vi "Tick.vi"(7 "error in (no error)":errorcluster) -> (5 "error out":errorcluster, 11 "seconds":dbl)   [LabVIEW 2026]
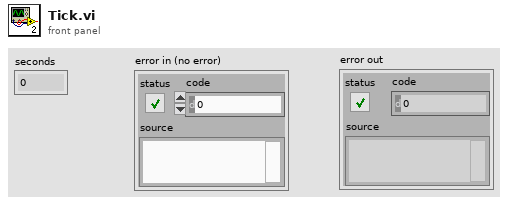
[diagram p1: front panel]
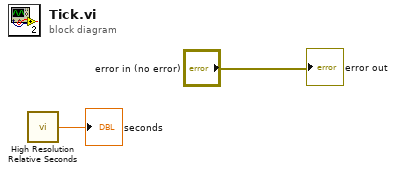
[diagram p0: block diagram]
diagram:
  n1 = call <vilib>:"High Resolution Relative Seconds.vi"() -> ("relative seconds"=→"seconds":dbl)
  "error out" <- "error in (no error)"
